vi "mqttTXdataQueueEnqueue.vi"(5 "data in":u8[](array[numeric]) format="%x", 11 "error in (no error)":errorcluster) -> (15 "error out":errorcluster)   [LabVIEW 2017]
uses:
  mqttTXdataQueueFunction.ctl
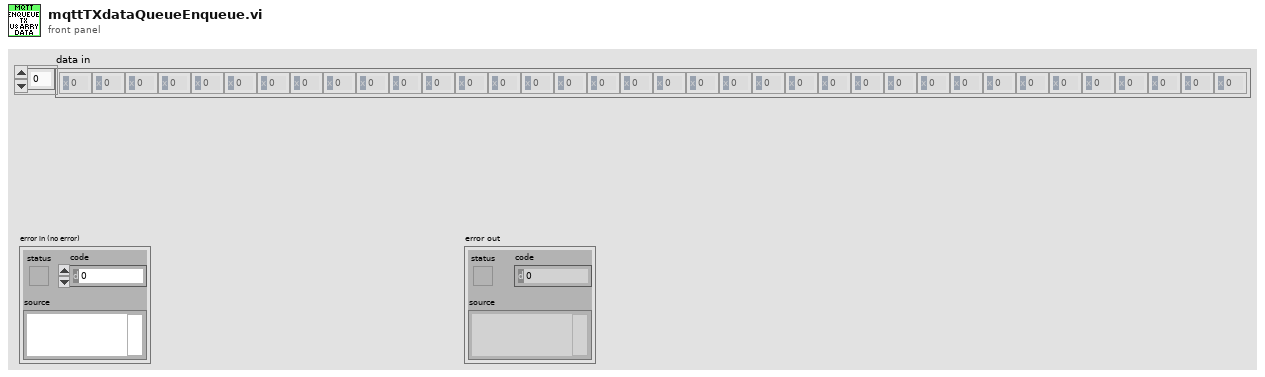
[diagram p1: front panel]
types:
  T1 = typedef "mqttTXdataQueueFunction.ctl" = enum16{"init", "deinit", "getQueue", "enqueue", "flushQueue"}
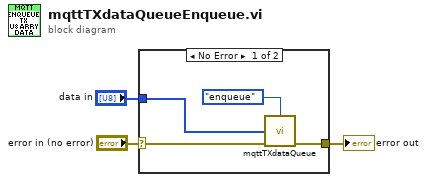
[diagram p0: block diagram]
diagram:
  n1 = case shown="No Error" "error in (no error)" {
    selector: "error in (no error)" -> [w7 w8]
    tunnel: [w4 w8] -> w2
    tunnel: "data in" -> [w6 _]
    frame No Error {
      n2 = call "mqttTXdataQueue.vi"("function"=mqttTXdataQueueFunction."enqueue", "telegram"=w6, "error in (no error)"=w7) -> ("error out"=w4:errorcluster)  [unwired: 10 in, 2 out]
    }
    frame Error {
    }
  }
  "error out" <- w2
